vi "Test Publish Packet.vi"() -> ()   [LabVIEW 2013]
uses:
  source/Control Packets/PUBLISH/PUBLISH.lvclass
  <vilib>/LabVIEW Open Source Project/Configuration Manager/Serializer/Serializer.lvclass
  source/Control Packets/ControlPacket/ControlPacket.lvclass/ControlPacket.ctl
  source/Control Packets/ControlPacket/ControlPacket.lvclass
panel:
  out "Complete Packet 2":bool
  out "data 2":dbl
  out "number (0 to 1) 2":dbl
  out "number (0 to 1)":dbl
  out "data":dbl
  out "Complete Packet":bool
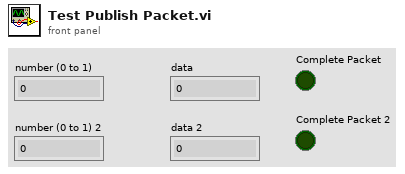
[diagram p1: front panel]
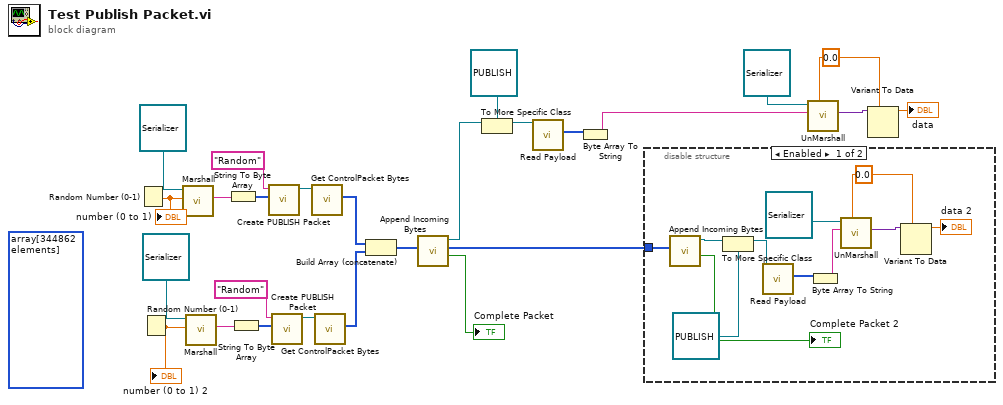
[diagram p0: block diagram]
diagram:
  w12 = 0.0
  (unwired) u8[] array[344862 elements] ("Incoming Packets")
  n1 = Random Number (0-1)() -> (number: 0 to 1=w24:dbl)
  "number (0 to 1)" <- w24
  n2 = Random Number (0-1)() -> (number: 0 to 1=w7:dbl)
  "number (0 to 1) 2" <- w7
  n3 = call-dynamic "Marshall.vi"("Variant"=w24, "Serializer in"=refnum<class "Serializer.lvclass"> refnum) -> ("String"=w26:string)  [unwired: 7 in, 2 out]
  n4 = call-dynamic "Marshall.vi"("Variant"=w7, "Serializer in"=refnum<class "Serializer.lvclass"> refnum) -> ("String"=w5:string)  [unwired: 7 in, 2 out]
  n5 = String To Byte Array(string=w26) -> (unsigned byte array=w18:u8[])
  n6 = String To Byte Array(string=w5) -> (unsigned byte array=w10:u8[])
  n7 = call "Create PUBLISH Packet.vi"("Payload"=w18, "Topic Name"="Random") -> ("PUBLISH"=w22:refnum<class "PUBLISH.lvclass">)  [unwired: 7 in, 2 out]
  n8 = call "Create PUBLISH Packet.vi"("Payload"=w10, "Topic Name"="Random") -> ("PUBLISH"=w9:refnum<class "PUBLISH.lvclass">)  [unwired: 7 in, 2 out]
  n9 = call "Get ControlPacket Bytes.vi"("ControlPacket"=w22) -> ("Bytes Stream"=w3:u8[])  [unwired: 8 in, 2 out]
  n10 = call "Get ControlPacket Bytes.vi"("ControlPacket"=w9) -> ("Bytes Stream"=w4:u8[])  [unwired: 8 in, 2 out]
  n11 = Build Array (concatenate)(w3, w4) -> (w2:u8[])
  n12 = call "Append Incoming Bytes.vi"("Incoming Packets"=w2) -> ("Complete Packet"=→"Complete Packet":bool, "Remaining Packets"=w1:u8[], "ControlPacket"=w20:refnum<class "ControlPacket.lvclass">)  [unwired: 7 in, 1 out]
  n13 = To More Specific Class(target class=refnum<class "PUBLISH.lvclass"> refnum ("PUBLISH.lvclass"), reference=w20) -> (specific class reference=w17:refnum<class "PUBLISH.lvclass">)  [unwired: 1 in, 1 out]
  n14 = call "Read Payload.vi"("ControlPacket in"=w17) -> ("Payload"=w15:u8[])  [unwired: 9 in, 1 out]
  n15 = Byte Array To String(unsigned byte array=w15) -> (string=w14:string)
  n16 = disable-structure shown="Enabled" {
    disable-tunnel: w1 -> [w37 _]
    frame Enabled {
      w31 = 0.0
      n17 = call "Append Incoming Bytes.vi"("Incoming Packets"=w37) -> ("Complete Packet"=→"Complete Packet 2":bool, "ControlPacket"=w35:refnum<class "ControlPacket.lvclass">)  [unwired: 7 in, 2 out]
      n18 = To More Specific Class(target class=refnum<class "PUBLISH.lvclass"> refnum ("PUBLISH.lvclass"), reference=w35) -> (specific class reference=w33:refnum<class "PUBLISH.lvclass">)  [unwired: 1 in, 1 out]
      n19 = call "Read Payload.vi"("ControlPacket in"=w33) -> ("Payload"=w34:u8[])  [unwired: 9 in, 1 out]
      n20 = Byte Array To String(unsigned byte array=w34) -> (string=w29:string)
      n21 = call-dynamic "UnMarshall.vi"("Type"=w31, "String"=w29, "Serializer in"=refnum<class "Serializer.lvclass"> refnum) -> ("Variant"=w30:variant)  [unwired: 6 in, 2 out]
      n22 = Variant To Data(type=w31, Variant=w30) -> (data=→"data 2":dbl)  [unwired: 1 in, 1 out]
    }
    frame Disabled {
    }
  }
  n23 = call-dynamic "UnMarshall.vi"("Type"=w12, "String"=w14, "Serializer in"=refnum<class "Serializer.lvclass"> refnum) -> ("Variant"=w13:variant)  [unwired: 6 in, 2 out]
  n24 = Variant To Data(type=w12, Variant=w13) -> (data=→"data":dbl)  [unwired: 1 in, 1 out]
